vi "Left - Open Tray.vi"(8 "error in (no error)":errorcluster, 10 "Ctl Refnum":refnum<vi>) -> (0 "error out":errorcluster)   [LabVIEW 2011, in "SlideEngine.lvclass"]
uses:
  SlideEngine.lvclass
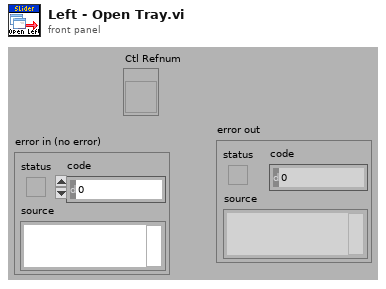
[diagram p1: front panel]
types:
  T1 = typedef "LVPositionTypeDef.ctl" = cluster{"Left":i32, "Top":i32}
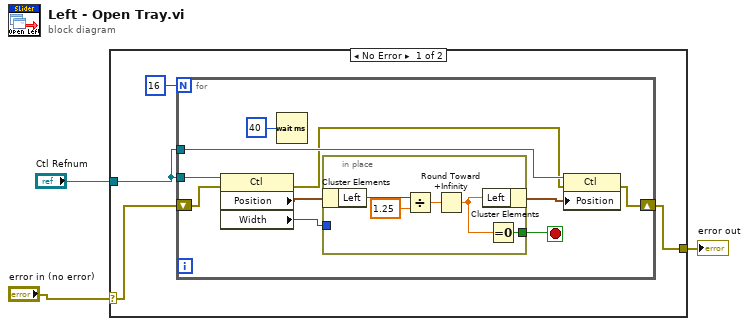
[diagram p0: block diagram]
diagram:
  n1 = case shown="No Error" "error in (no error)" {
    selector: "error in (no error)" -> [w5 w23]
    tunnel: "Ctl Refnum" -> [w6 _]
    tunnel: [w4 w23] -> w1
    frame No Error {
      n2 = for {
        N: 16 -> [_]
        tunnel: w6 -> [w13]
        tunnel: w6 -> [w12]
        shift-right: [w9] -> w4
        shift-left: w5 -> [w11]
        stop <- w8 stop-if-true
        n3 = property on="Property Node" class="Ctl"(reference=w13, error in=w11) -> (error out=w10:errorcluster, "Position"=w17:T1, "Width"=w14:u32)  [unwired: 1 out]
        n4 = Wait (ms)(milliseconds to wait=u32 40) -> ()  [unwired: 1 out]
        n5 = in-place {
          in-place-border: w14 -> [_]
          in-place-border: [w18] -> w8
          n6 = in-place-cluster #1(w17) -> ("Left"=w22:i32)
          n7 = Divide(x=w22, y=1.25) -> (x/y=w21:dbl)
          n8 = Round Toward +Infinity(x=w21) -> (ceil(x): smallest int >= x=w19:dbl)
          n9 = in-place-cluster #1("Left"=w19) -> (w16:T1)
          n10 = Equal To 0?(x=w19) -> (x = 0?=w18:bool)
        }
        n11 = property on="Property Node" class="Ctl"(reference=w12, error in=w10, "Position"=w16) -> (error out=w9:errorcluster)  [unwired: 1 out]
      }
    }
    frame Error {
    }
  }
  "error out" <- w1
